vi "Centrifuge Settings Dialog.vi"(8 "error in (no error)":errorcluster, 10 "Message Queues":T8, 11 "Pump Module State Cluster In":T1={"Centrifuge Module Config"={"GUID"="", "Drop Coords"={"Horizontal"=0, "Vertical"=0}, "Process Name"="", "User name"="", "Queue Name"="", "Settings"={"Cycle Period"=500.0, "Manual Entry"=0.0, "Output Device"=enum."Default", "EPOS4 Settings"={"VISA resource name"="", "axis"={"keyHandle"=1, "nodeId"=1}, "Simulated?"=TRUE}}, "Load Count"=0}, "State"=enum."Idle", "Start Time"=timestamp(0 s since 1904-01-01), "Current Time"=timestamp(0 s since 1904-01-01), "First Iteration"=FALSE, "Data"={"Centrifuge Speed"=0.0}, "Process Name"="", "Centrifuge On?"=FALSE}) -> (0 "error out":errorcluster, 1 "Cancelled?":bool=TRUE, 2 "UI Refresh Needed?":bool, 3 "Centrifuge Module Config Out":T2={"GUID"="", "Drop Coords"={"Horizontal"=0, "Vertical"=0}, "Process Name"="", "User name"="", "Queue Name"="", "Settings"={"Cycle Period"=0.0, "Manual Entry"=0.0, "Output Device"=enum."Default", "EPOS4 Settings"={"VISA resource name"="", "axis"={"keyHandle"=1, "nodeId"=1}, "Simulated?"=FALSE}}, "Load Count"=0})   [LabVIEW 2018, in "Centrifuge Module.lvlib"]
doc: "Dialog for selecting user specified settings."
uses:
  Centrifuge Module.lvlib
  Centrifuge Dialog Config and Start Stop Buttons.ctl
  EPOS4/Controls/Device Selection.ctl
  EPOS4/Controls/EPOS Communication Settings.ctl
  All Message Queues.ctl
  support/Message Queue/Message Cluster.ctl
  Centrifuge Module Config Cluster.ctl
  <vilib>/Utility/miscctls.llb/LVPoint32TypeDef.ctl
  Centrifuge Module Settings Cluster.ctl
  Centrifuge Module State Cluster.ctl
  Measure Instrument/State Enum.ctl
  Measure Instrument/PID 2 Output Enum.ctl
  support/Message Queue/Enqueue Message (Single).vi
  <vilib>/Utility/xml.llb/Write to XML File(string).vi
  Settings/Settings.lvlib
  support/Support Library.lvlib
  support/Message Queue/Message Queue.lvlib
  EPOS4/EPOS4.lvlib
  Measure Instrument/Feed Module Engine.lvlib
panel:
  in  "Module Name":string
  in  "Centrifuge Settings":T9
  in  "Cancel Button":bool
  in  "OK Button":bool
  # "Non visible portion of dialog (needed for connector pane)."
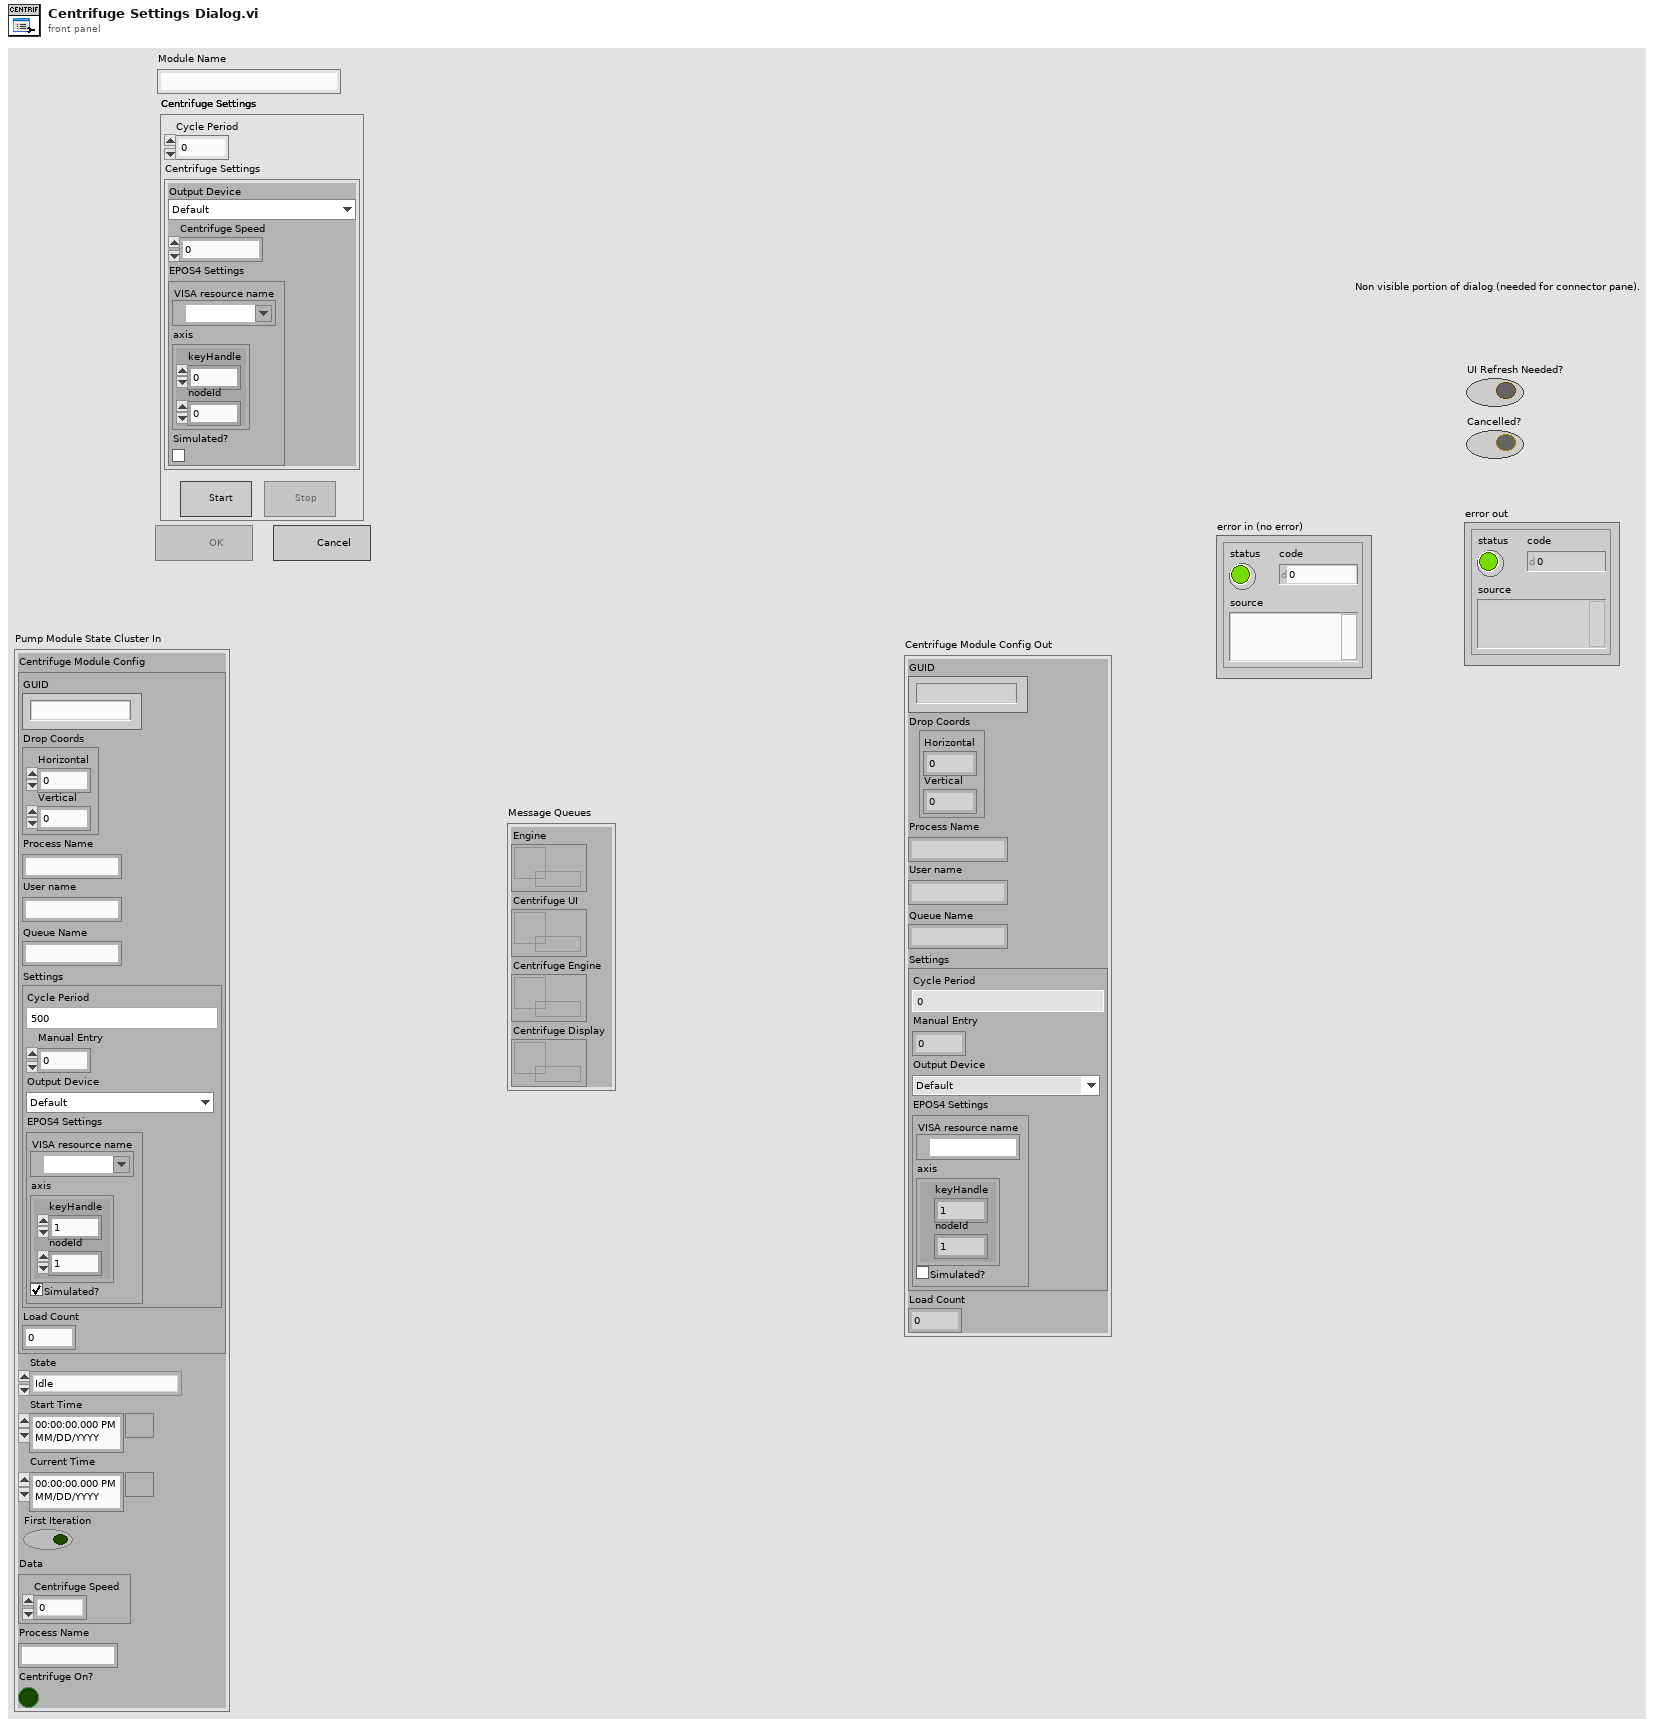
[diagram p1: front panel]
types:
  T1 = typedef "Centrifuge Module.lvlib/Centrifuge Module State Cluster.ctl" = cluster{"Centrifuge Module Config":T2, "State":T7, "Start Time":timestamp, "Current Time":timestamp, "First Iteration":bool, "Data":cluster{"Centrifuge Speed":dbl}, "Process Name":string, "Centrifuge On?":bool}
  T2 = typedef "Centrifuge Module.lvlib/Centrifuge Module Config Cluster.ctl" = cluster{"GUID":string, "Drop Coords":T3, "Process Name":string, "User name":string, "Queue Name":string, "Settings":T4, "Load Count":i32}
  T3 = typedef "LVPoint32TypeDef.ctl" = cluster{"Horizontal":i32, "Vertical":i32}
  T4 = typedef "Centrifuge Module.lvlib/Centrifuge Module Settings Cluster.ctl" = cluster{"Cycle Period":dbl, "Manual Entry":dbl, "Output Device":T5, "EPOS4 Settings":T6}
  T5 = typedef "Device Selection.ctl" = enum16{"Default", "EPOS4"}
  T6 = typedef "EPOS4.lvlib/EPOS Communication Settings.ctl" = cluster{"VISA resource name":refnum<visa-resource-name>, "axis":cluster{"keyHandle":u32, "nodeId":u16}, "Simulated?":bool}
  T7 = typedef "Feed Module.lvlib/Feed Module Engine.lvlib/State Enum.ctl" = enum16{"Measuring", "Idle", "Paused"}
  T8 = typedef "Centrifuge Module.lvlib/All Message Queues.ctl" = cluster{"Engine":refnum<queue>, "Centrifuge UI":refnum<queue>, "Centrifuge Engine":refnum<queue>, "Centrifuge Display":refnum<queue>}
  T9 = typedef "Centrifuge Module.lvlib/Centrifuge Dialog Config and Start Stop Buttons.ctl" = cluster{"Cycle Period":dbl, "Centrifuge Settings":cluster{"Output Device":T5, "Pump %":dbl, "EPOS4 Settings":T6}, "Stop":bool, "Start":bool}
  T10 = typedef "PID 2 Output Enum.ctl" = enum16{"Default", "Ismatec ISM 4308", "Ismatec ISM 831C", "Masterflex 7550-30", "VICI M6", "VICI M50", "Tacmina QI", "KNF SIMDOS", "ASIA Type C", "FLOM UI-22-11", "SSI PR/LD", "SSI P40", "Masterflex 75211-70"}
  T11 = enum8{"Enabled", "Disabled", "Disabled and Grayed Out"}
  T12 = cluster{"Output Device":T5, "Pump %":dbl, "EPOS4 Settings":T6}
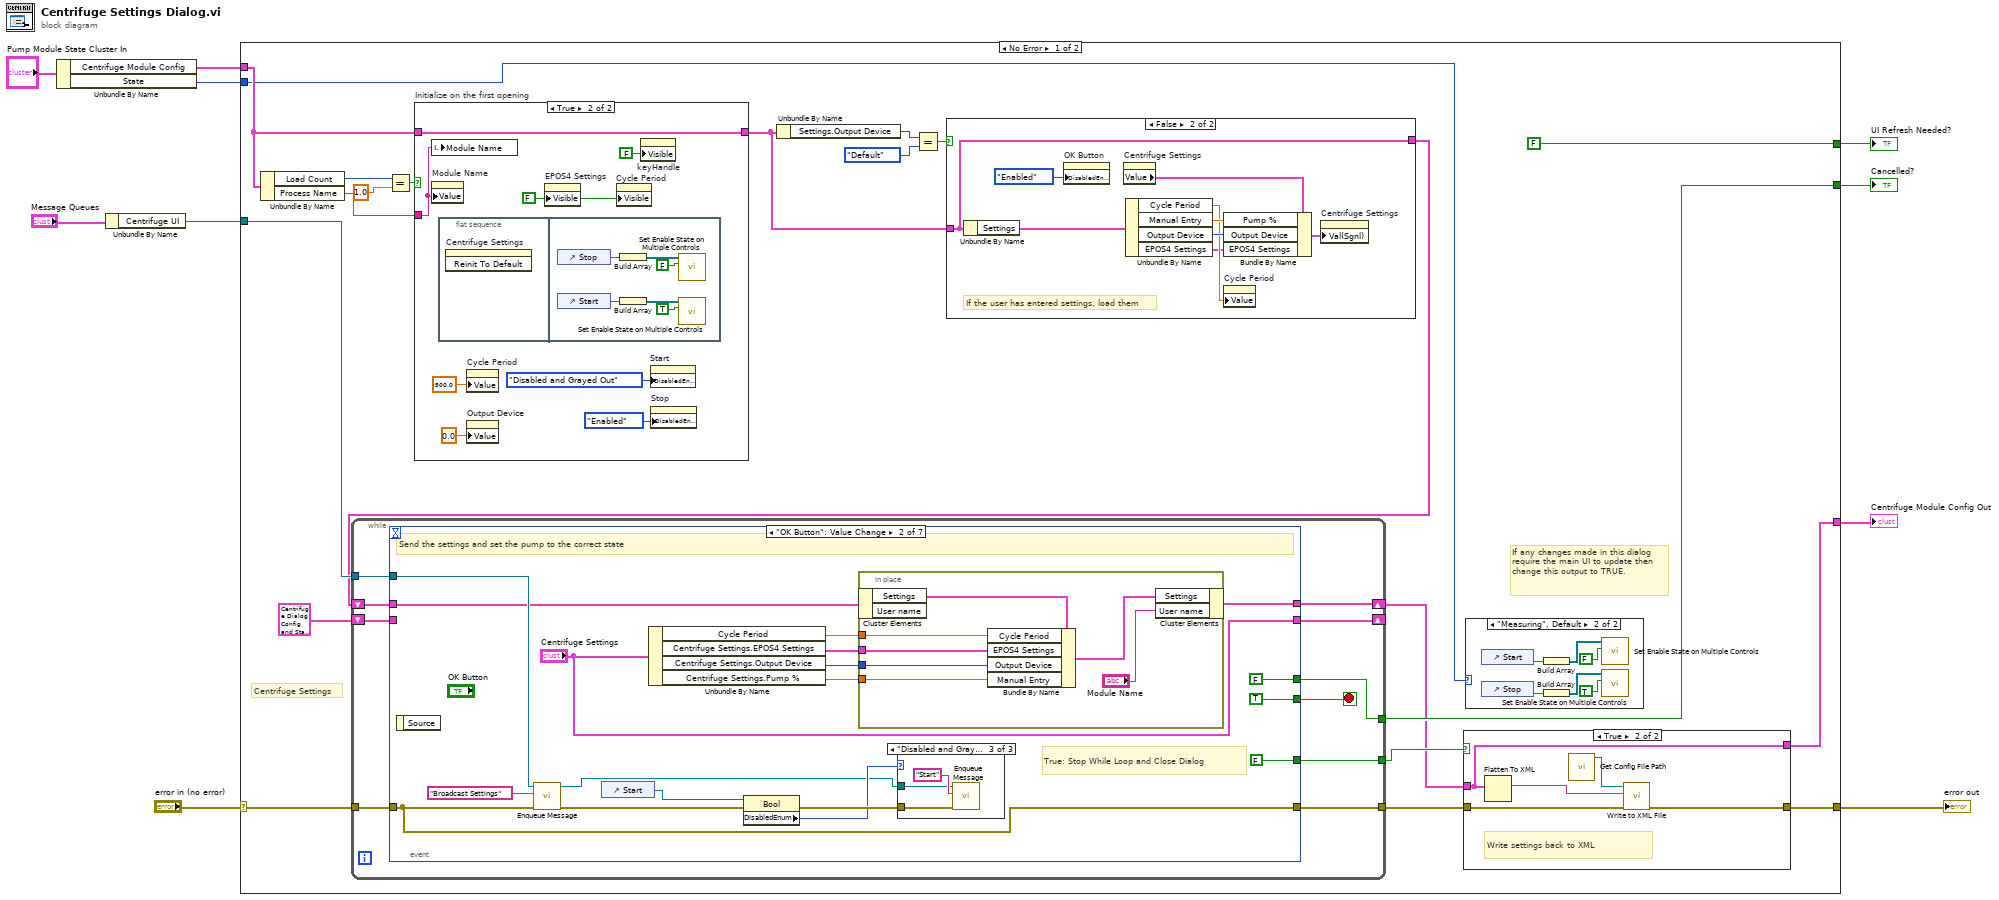
[diagram p0: block diagram]
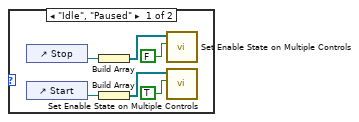
[diagram p2: hidden frame]
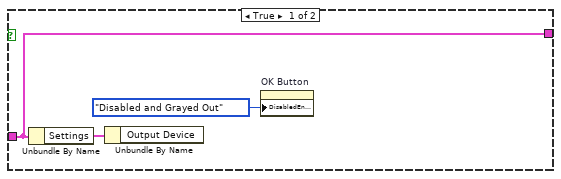
[diagram p3: hidden frame]
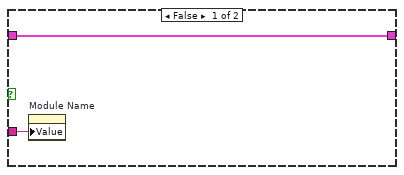
[diagram p4: hidden frame]
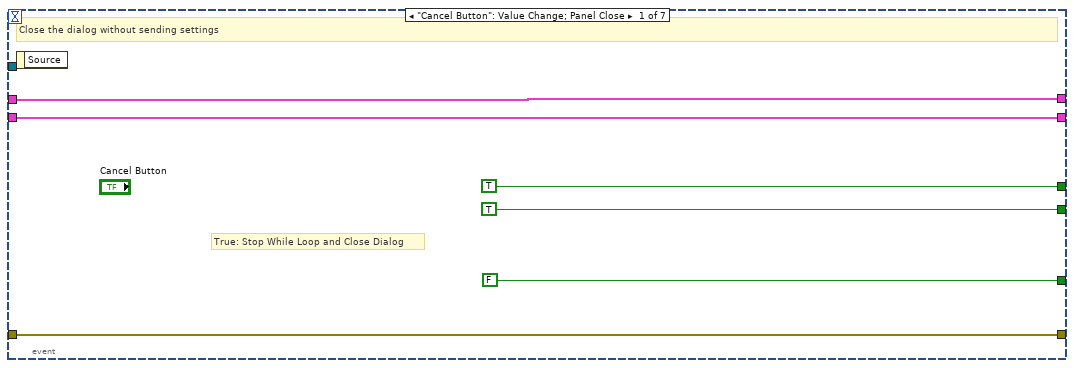
[diagram p5: hidden frame]
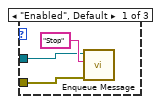
[diagram p6: hidden frame]
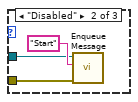
[diagram p7: hidden frame]
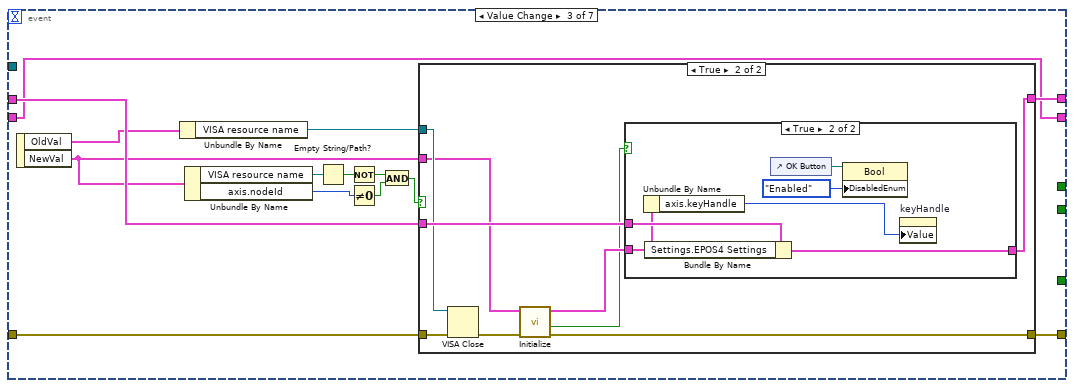
[diagram p8: hidden frame]
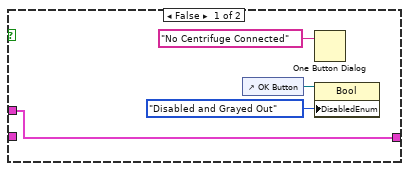
[diagram p10: hidden frame]
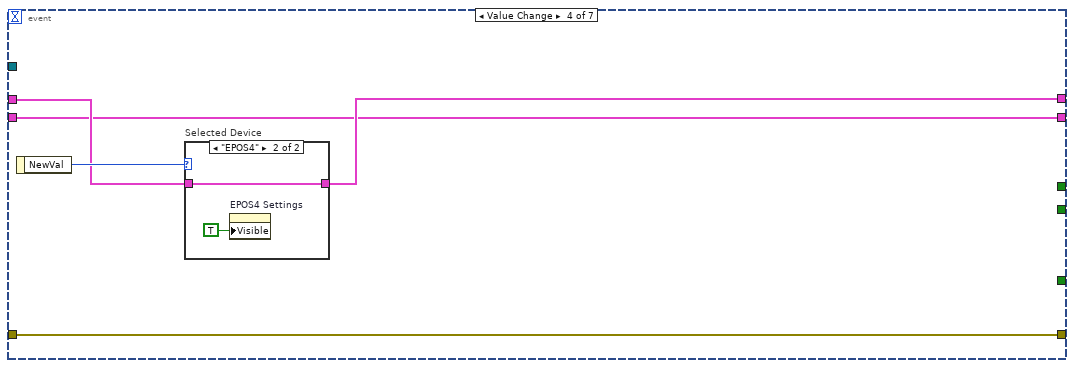
[diagram p11: hidden frame]
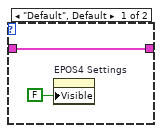
[diagram p12: hidden frame]
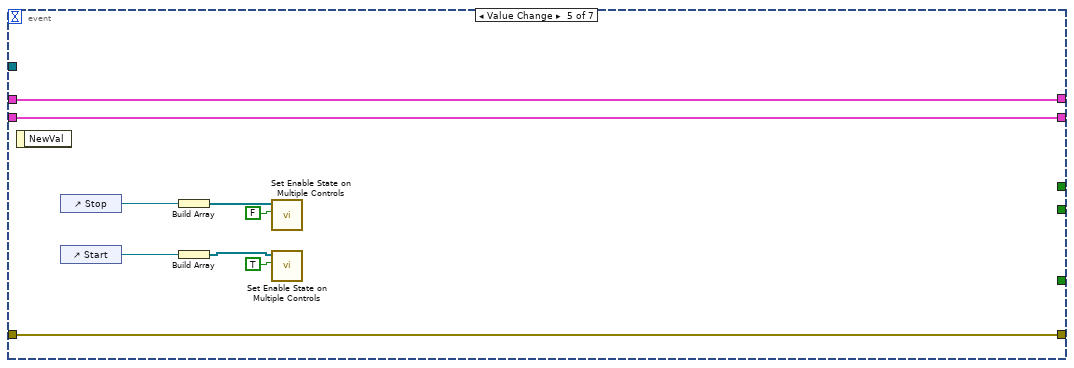
[diagram p13: hidden frame]
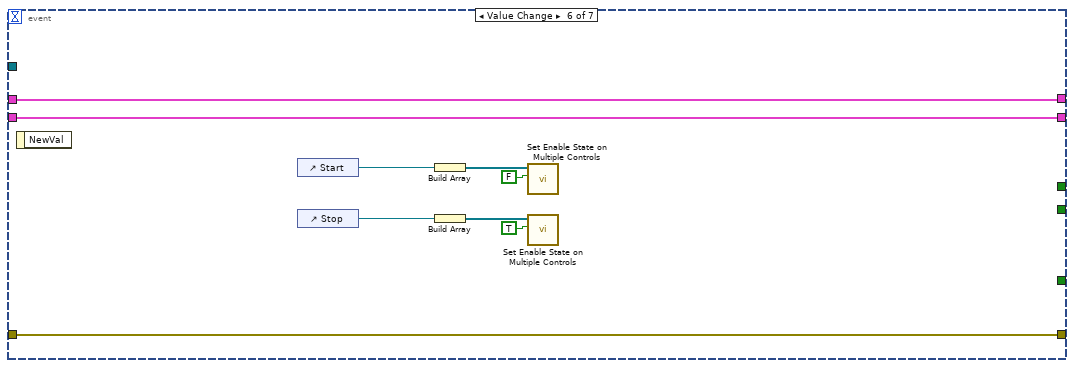
[diagram p14: hidden frame]
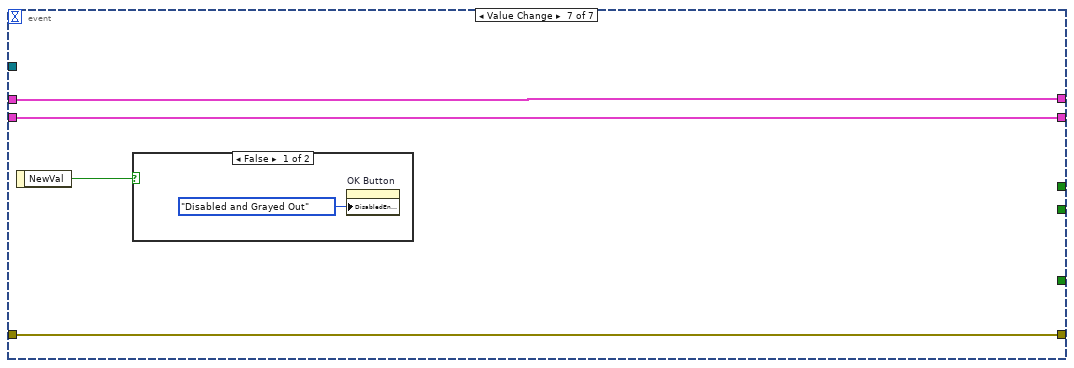
[diagram p15: hidden frame]
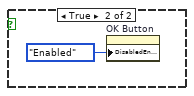
[diagram p16: hidden frame]
diagram:
  n1 = Unbundle By Name("Pump Module State Cluster In") -> ("Centrifuge Module Config"=w2:T2, "State"=w1:T7)
  n2 = Unbundle By Name("Message Queues") -> ("Centrifuge UI"=w7:refnum<queue>)
  n3 = case shown="No Error" "error in (no error)" {
    selector: "error in (no error)" -> [w26 w198]
    tunnel: [w28 w198] -> w10
    tunnel: w2 -> [w25 w196]
    tunnel: [w29 w196] -> w4
    tunnel: [FALSE ("UI Refresh Needed?") _] -> w9
    tunnel: [w30 TRUE ("UI Refresh Needed?")] -> w8
    tunnel: w7 -> [w27 _]
    tunnel: w1 -> [w24 _]
    frame No Error {
      # "Centrifuge Settings"
      # "If any changes made in this dialog require the main UI to update then change this output to TRUE."
      n4 = Unbundle By Name(w25) -> ("Load Count"=w23:i32, "Process Name"=w13:string)
      n5 = Equal?(x=w23, y=1.0) -> (x = y?=w21:bool)
      n6 = case "Initialize on the first opening" shown="True" w21 {
        tunnel: w25 -> [w57 w65]
        tunnel: [w57 w65] -> w17
        tunnel: w13 -> [w56 w64]
        frame False {
          n7 = property on="Module Name" class="Str"("Value"=w56) -> ()  [unwired: 2 in, 2 out]
        }
        frame True {
          w61 = FALSE ("Visible")
          n8 = local write "Module Name"(w64) -> ()
          n9 = property on="Module Name" class="Str"("Value"=w64) -> ()  [unwired: 2 in, 2 out]
          n10 = flat-sequence {
            frame #0 {
              n11 = invoke on="Centrifuge Settings" class="Clust" method="Reinit To Default"() -> ()  [unwired: 3 in, 3 out]
            }
            frame #1 {
              n12 = control-ref of="Stop"() -> (w68:refnum<vi>)
              n13 = control-ref of="Start"() -> (w71:refnum<vi>)
              n14 = Build Array(w68) -> (w67:refnum<vi>[])
              n15 = Build Array(w71) -> (w70:refnum<vi>[])
              n16 = call "Set Enable State on Multiple Controls.vi"("Enable?"=FALSE, "Controls"=w67) -> ()  [unwired: 10 in]
              n17 = call "Set Enable State on Multiple Controls.vi"("Enable?"=TRUE, "Controls"=w70) -> ()  [unwired: 10 in]
            }
          }
          n18 = property on="Cycle Period" class="DigNum (strict)"("Value"=500.0) -> ()  [unwired: 2 in, 2 out]
          n19 = property on="Output Device" class="Enum (strict)"("Value"=0.0) -> ()  [unwired: 2 in, 2 out]
          n20 = property on="EPOS4 Settings" class="Clust (strict)"("Visible"=w61) -> ()  [unwired: 2 in, 2 out]
          n21 = property on="Cycle Period" class="DigNum (strict)"("Visible"=w61) -> ()  [unwired: 2 in, 2 out]
          n22 = property on="keyHandle" class="DigNum (strict)"("Visible"=FALSE) -> ()  [unwired: 2 in, 2 out]
          n23 = property on="Start" class="Bool"("DisabledEnum"=T11."Disabled and Grayed Out" ("Disabled")) -> ()  [unwired: 2 in, 2 out]
          n24 = property on="Stop" class="Bool"("DisabledEnum"=T11."Enabled" ("Disabled")) -> ()  [unwired: 2 in, 2 out]
        }
      }
      n25 = Unbundle By Name(w17) -> ("Settings.Output Device"=w15:T5)
      n26 = Equal?(x=w15, y=PID_2_Output_Enum."Default" ("Settings.Output Device")) -> (x = y?=w14:bool)
      n27 = case shown="False" w14 {
        tunnel: w17 -> [w45 w52]
        tunnel: [w45 w52] -> w18
        frame True {
          n28 = Unbundle By Name(w45) -> ("Settings"=w46:T4)
          n29 = Unbundle By Name(w46) -> ()  [unwired: 1 out]
          n30 = property on="OK Button" class="Bool"("DisabledEnum"=T11."Disabled and Grayed Out" ("Disabled")) -> ()  [unwired: 2 in, 2 out]
        }
        frame False {
          # "If the user has entered settings, load them"
          n31 = Unbundle By Name(w52) -> ("Settings"=w54:T4)
          n32 = property on="OK Button" class="Bool"("DisabledEnum"=T11."Enabled" ("Disabled")) -> ()  [unwired: 2 in, 2 out]
          n33 = property on="Centrifuge Settings" class="Clust (strict)"() -> ("Value"=w48:T12)  [unwired: 2 in, 2 out]
          n34 = Unbundle By Name(w54) -> ("Cycle Period"=w49:dbl, "Manual Entry"=w51:dbl, "Output Device"=w50:T5, "EPOS4 Settings"=w47:T6)
          n35 = Bundle By Name(cluster=w48, "Pump %"=w51, "Output Device"=w50, "EPOS4 Settings"=w47) -> (w55:T12)
          n36 = property on="Cycle Period" class="DigNum (strict)"("Value"=w49) -> ()  [unwired: 2 in, 2 out]
          n37 = property on="Centrifuge Settings" class="Clust"("Val(Sgnl)"=w55) -> ()  [unwired: 2 in, 2 out]
        }
      }
      n38 = while {
        tunnel: [w81] -> w20
        tunnel: [w79] -> w30
        tunnel: w27 -> [w77]
        tunnel: w26 -> [w76]
        shift-right: [w78] -> w19
        shift-left: w18 -> [w75]
        shift-right: [w74] -> _
        shift-left: T9 {"Cycle Period"=0.0, "Centrifuge Settings"={"Output Device"=enum."Default", "Pump %"=0.0, "EPOS4 Settings"={"VISA resource name"="", "axis"={"keyHandle"=0, "nodeId"=1}, "Simulated?"=FALSE}}, "Stop"=FALSE, "Start"=FALSE} ("Centrifuge Settings+buttons") -> [w73]
        tunnel: [w72] -> w11
        stop <- w80 stop-if-true
        n39 = event shown="[1] \"OK Button\": Value Change" {
          selector: _ -> [_ _ _ _ _ _ _]
          dyn-events: _ -> [_ _ _ _ _ _ _]
          timeout: _ -> [_ _ _ _ _ _ _]
          tunnel: [FALSE ("UI Refresh Needed?") FALSE ("UI Refresh Needed?") _ _ _ _ _] -> w81
          tunnel: [TRUE TRUE _ _ _ _ _] -> w80
          tunnel: [TRUE ("UI Refresh Needed?") FALSE ("UI Refresh Needed?") _ _ _ _ _] -> w79
          tunnel: w75 -> [w84 w91 w135 w160 w169 w178 w187]
          tunnel: [w84 w90 w134 w159 w169 w178 w187] -> w78
          tunnel: w77 -> [_ w102 _ _ _ _ _]
          tunnel: w76 -> [w82 w101 w133 w157 w166 w175 w185]
          tunnel: [w83 "Centrifuge Settings" w132 w158 w168 w177 w186] -> w74
          tunnel: w73 -> [w83 _ w132 w158 w168 w177 w186]
          tunnel: [w82 w101 w131 w157 w166 w175 w185] -> w72
          event "Cancel Button": Value Change; Panel Close {
            # "True: Stop While Loop and Close Dialog"
            # "Close the dialog without sending settings"
            n40 = event-data() -> ()  [unwired: 1 in, 1 out]
          }
          event "OK Button": Value Change {
            # "True: Stop While Loop and Close Dialog"
            # "Send the settings and set the pump to the correct state"
            n41 = event-data() -> ()  [unwired: 1 in, 1 out]
            n42 = call-poly "Enqueue Message.vi"("error in (no error)"=w101, "Message"="Broadcast Settings", "Message Queue"=w102) -> ("error out"=w93:errorcluster, "dup Message Queue"=w92:refnum<queue>)  [unwired: 7 in]
            n43 = control-ref of="Start"() -> (w96:refnum<vi>)
            n44 = Unbundle By Name("Centrifuge Settings") -> ("Cycle Period"=w88:dbl, "Centrifuge Settings.EPOS4 Settings"=w100:T6, "Centrifuge Settings.Output Device"=w89:T5, "Centrifuge Settings.Pump %"=w99:dbl)
            n45 = property class="Bool"(reference=w96, error in=w93) -> (error out=w97:errorcluster, "DisabledEnum"=w95:T11)  [unwired: 1 out]
            n46 = in-place {
              in-place-border: w100 -> [w112]
              in-place-border: w99 -> [w108]
              in-place-border: w89 -> [w109]
              in-place-border: w88 -> [w107]
              n47 = in-place-cluster #1(w91) -> ("Settings"=w110:T4)  [unwired: 1 out]
              n48 = Bundle By Name(cluster=w110, "Cycle Period"=w107, "EPOS4 Settings"=w112, "Output Device"=w109, "Manual Entry"=w108) -> (w111:T4)
              n49 = in-place-cluster #1("Settings"=w111, "User name"="Module Name") -> (w90:T2)
            }
            n50 = case shown="\"Disabled and Grayed Out\"" w95 {
              tunnel: w97 -> [w114 w117 w120]
              tunnel: w92 -> [w113 w116 w119]
              frame "Enabled", Default {
                n51 = call-poly "Enqueue Message.vi"("error in (no error)"=w114, "Message"="Stop", "Message Queue"=w113) -> ()  [unwired: 7 in, 2 out]
              }
              frame "Disabled" {
                n52 = call-poly "Enqueue Message.vi"("error in (no error)"=w117, "Message"="Start", "Message Queue"=w116) -> ()  [unwired: 7 in, 2 out]
              }
              frame "Disabled and Grayed Out" {
                n53 = call-poly "Enqueue Message.vi"("error in (no error)"=w120, "Message"="Start", "Message Queue"=w119) -> ()  [unwired: 7 in, 2 out]
              }
            }
          }
          event Value Change {
            n54 = event-data() -> ("OldVal"=w130:T6, "NewVal"=w128:T6)  [unwired: 1 in]
            n55 = Unbundle By Name(w130) -> ("VISA resource name"=w129:refnum<visa-resource-name>)
            n56 = Unbundle By Name(w128) -> ("VISA resource name"=w126:refnum<visa-resource-name>, "axis.nodeId"=w127:u16)
            n57 = Empty String/Path?(string/path=w126) -> (empty?=w125:bool)
            n58 = Not(x=w125) -> (.not. x?=w124:bool)
            n59 = Not Equal To 0?(x=w127) -> (x != 0?=w123:bool)
            n60 = And(x=w124, y=w123) -> (x .and. y?=w122:bool)
            n61 = case shown="True" w122 {
              tunnel: w135 -> [w137 w146]
              tunnel: [w137 w145] -> w134
              tunnel: w133 -> [w136 w144]
              tunnel: [w136 w140] -> w131
              tunnel: w129 -> [_ w139]
              tunnel: w128 -> [_ w138]
              frame False {
              }
              frame True {
                n62 = VISA Close(VISA resource name=w139, error in (no error)=w144) -> (error out=w143:errorcluster)
                n63 = call "Initialize.vi"("error in (no error)"=w143, "EPOS4 Settings In"=w138) -> ("error out"=w140:errorcluster, "Initialized"=w141:bool, "EPOS4 Settings Out"=w142:T6)  [unwired: 6 in, 1 out]
                n64 = case shown="True" w141 {
                  tunnel: w142 -> [_ w152]
                  tunnel: w146 -> [w150 w156]
                  tunnel: [w150 w155] -> w145
                  frame False {
                    n65 = control-ref of="OK Button"() -> (w148:refnum<vi>)
                    n66 = One Button Dialog(message="No Centrifuge Connected") -> ()  [unwired: 1 in, 1 out]
                    n67 = property class="Bool"(reference=w148, "DisabledEnum"=T11."Disabled and Grayed Out" ("Disabled")) -> ()  [unwired: 1 in, 2 out]
                  }
                  frame True {
                    n68 = Unbundle By Name(w152) -> ("axis.keyHandle"=w151:u32)
                    n69 = Bundle By Name(cluster=w156, "Settings.EPOS4 Settings"=w152) -> (w155:T2)
                    n70 = control-ref of="OK Button"() -> (w153:refnum<vi>)
                    n71 = property class="Bool"(reference=w153, "DisabledEnum"=T11."Enabled" ("Disabled")) -> ()  [unwired: 1 in, 2 out]
                    n72 = property on="keyHandle" class="DigNum (strict)"("Value"=w151) -> ()  [unwired: 2 in, 2 out]
                  }
                }
              }
            }
          }
          event Value Change {
            n73 = event-data() -> ("NewVal"=w161:T5)  [unwired: 1 in]
            n74 = case "Selected Device" shown="\"EPOS4\"" w161 {
              tunnel: w160 -> [w162 w165]
              tunnel: [w162 w165] -> w159
              frame "Default", Default {
                n75 = property on="EPOS4 Settings" class="Clust (strict)"("Visible"=FALSE) -> ()  [unwired: 2 in, 2 out]
              }
              frame "EPOS4" {
                n76 = property on="EPOS4 Settings" class="Clust (strict)"("Visible"=TRUE) -> ()  [unwired: 2 in, 2 out]
              }
            }
          }
          event Value Change {
            n77 = event-data() -> ()  [unwired: 1 in, 1 out]
            n78 = control-ref of="Stop"() -> (w170:refnum<vi>)
            n79 = control-ref of="Start"() -> (w167:refnum<vi>)
            n80 = Build Array(w170) -> (w172:refnum<vi>[])
            n81 = Build Array(w167) -> (w174:refnum<vi>[])
            n82 = call "Set Enable State on Multiple Controls.vi"("Enable?"=FALSE, "Controls"=w172) -> ()  [unwired: 10 in]
            n83 = call "Set Enable State on Multiple Controls.vi"("Enable?"=TRUE, "Controls"=w174) -> ()  [unwired: 10 in]
          }
          event Value Change {
            n84 = event-data() -> ()  [unwired: 1 in, 1 out]
            n85 = control-ref of="Start"() -> (w176:refnum<vi>)
            n86 = control-ref of="Stop"() -> (w179:refnum<vi>)
            n87 = Build Array(w176) -> (w181:refnum<vi>[])
            n88 = Build Array(w179) -> (w183:refnum<vi>[])
            n89 = call "Set Enable State on Multiple Controls.vi"("Enable?"=FALSE, "Controls"=w181) -> ()  [unwired: 10 in]
            n90 = call "Set Enable State on Multiple Controls.vi"("Enable?"=TRUE, "Controls"=w183) -> ()  [unwired: 10 in]
          }
          event Value Change {
            n91 = event-data() -> ("NewVal"=w184:bool)  [unwired: 1 in]
            n92 = case shown="False" w184 {
              frame False {
                n93 = property on="OK Button" class="Bool"("DisabledEnum"=T11."Disabled and Grayed Out" ("Disabled")) -> ()  [unwired: 2 in, 2 out]
              }
              frame True {
                n94 = property on="OK Button" class="Bool"("DisabledEnum"=T11."Enabled" ("Disabled")) -> ()  [unwired: 2 in, 2 out]
              }
            }
          }
        }
      }
      n95 = case shown="True" w20 {
        tunnel: w19 -> [w190 w192]
        tunnel: [_ w193] -> w28
        tunnel: [w190 w192] -> w29
        tunnel: w11 -> [_ w191]
        frame False {
        }
        frame True {
          # "Write settings back to XML"
          n96 = Flatten To XML(anything=w192) -> (xml string=w194:string)
          n97 = call "Get Config File Path.vi"() -> ("XML File Path"=w195:path)  [unwired: 10 in, 1 out]
          n98 = call-poly <vilib>:"Write to XML File.vi"("error in (no error)"=w191, "XML Input"=w194, "XML File Path"=w195) -> ("error out"=w193:errorcluster)  [unwired: 6 in, 2 out]
        }
      }
      n99 = case shown="\"Measuring\", Default" w24 {
        frame "Idle", "Paused" {
          n100 = control-ref of="Stop"() -> (w32:refnum<vi>)
          n101 = control-ref of="Start"() -> (w34:refnum<vi>)
          n102 = Build Array(w32) -> (w36:refnum<vi>[])
          n103 = Build Array(w34) -> (w33:refnum<vi>[])
          n104 = call "Set Enable State on Multiple Controls.vi"("Enable?"=FALSE, "Controls"=w36) -> ()  [unwired: 10 in]
          n105 = call "Set Enable State on Multiple Controls.vi"("Enable?"=TRUE, "Controls"=w33) -> ()  [unwired: 10 in]
        }
        frame "Measuring", Default {
          n106 = control-ref of="Start"() -> (w38:refnum<vi>)
          n107 = control-ref of="Stop"() -> (w39:refnum<vi>)
          n108 = Build Array(w38) -> (w42:refnum<vi>[])
          n109 = Build Array(w39) -> (w40:refnum<vi>[])
          n110 = call "Set Enable State on Multiple Controls.vi"("Enable?"=FALSE, "Controls"=w42) -> ()  [unwired: 10 in]
          n111 = call "Set Enable State on Multiple Controls.vi"("Enable?"=TRUE, "Controls"=w40) -> ()  [unwired: 10 in]
        }
      }
    }
    frame Error {
    }
  }
  "UI Refresh Needed?" <- w9
  "error out" <- w10
  "Cancelled?" <- w8
  "Centrifuge Module Config Out" <- w4
